vi "ui--test plot updates.vi"() -> ()   [LabVIEW 2021]
doc: "test the output of the theme on a graph and chart\n\n<b>Code Developed By:</b>\nTechnology Service Corporation\nwww.tsc.com/atcs\n\nDeveloper:\nDaniel Coons"
uses:
  <vilib>/numeric/Random Number (Range) DBL.vi
panel:
  out "Waveform Graph 2":dbl[][](graph)=[[0.13306085440791815, 0.0879688901503013, 0.036775389853692886, 0.6532669979114305, 0.08472829522034431, 0.9983087206518939, 0.7170974439775832, 0.09862926455924459, 0.9104404133169357, 0.0033720393869565157, 0.3438860221523703, 0.09569147282292523, 0.05190666424335655, 0.24694252161785646, 0.5168863730093075, 0.26831134492038067, 0.8230969685646516, 0.9814472257906978, 0.2272061024550942, 0.8098917477502172, 0.887589550084189, 0.6100626174511069, 0.96603126360236, 0.9151131295841366, 0.7482899830981327, 0.2780702935515085, 0.4086091237019789, 0.5812795207762955, 0.7774140578159758, 0.7741649634708238, 0.6857088358139753, 0.8553493754163002, 0.827686972367776, 0.2529298655163781, 0.4874874814367782, 0.5367329241411547, 0.41191999774024723, 0.9360704793200025, 0.8481368597935868, 0.5851233104174891, 0.7460626166357829, 0.7675282163169203, 0.5941383079043361, 0.6084437811903307, 0.9137270207566848, 0.14164206553644543, 0.944367703009636, 0.9882229095650765, 0.12807404389957888, 0.10166795257813277, 0.32112247869774735, 0.5621551625675485, 0.7091308394444604, 0.6473377689678865, 0.007821979537185886, 0.8113619812952195, 0.8073576350852725, 0.08930872921975874, 0.14986848733562108, 0.011921153237574034, 0.570553517421061, 0.377967728590463, 0.04482355518779935, 0.3186424001717114, 0.21330456282949317, 0.0454940725453894, 0.5821532512218817, 0.15991602882719103, 0.5719089521252518, 0.7776511172742474, 0.4787019383389124, 0.09976918045663452, 0.18257053533382273, 0.5464087033728721, 0.7482146674486345, 0.7493376528505136, 0.8963704778416384, 0.7063016502139434, 0.15944801725401514, 0.847500088853314, 0.17171175112658021, 0.14952470286069142, 0.15221036496154827, 0.10203582642171849, 0.6420353678306143, 0.4906006710065236, 0.2651490386034048, 0.06996255442612176, 0.4658855102620627, 0.5430459637216143, 0.744480966535523, 0.027436968629737102, 0.2562650988536652, 0.25014985041664684, 0.1804990531180204, 0.6957082808752657, 0.41848772122628874, 0.24793827529423518, 0.8451613763305086, 0.27204098993248893], [2.250567331065164, 2.155222595371875, 2.2912157636499053, 2.635194602081454, 2.0113751602913768, 2.7614535130644526, 2.192032474109693, 2.5440494750975704, 2.648149659054945, 2.4445680167950696, 2.216467853336293, 2.873700551200666, 2.082048417331531, 2.2564812644354224, 2.8276488760055103, 2.9029889347562903, 2.8000502636985525, 2.91643317675736, 2.9143263543098397, 2.018791563346438, 2.6447330992967113, 2.6591634333013783, 2.4422995021207727, 2.0507560523333925, 2.173974032844874, 2.0288400085476557, 2.736724222763875, 2.1594821423701753, 2.0884083642674853, 2.8437861581589017, 2.594905434692701, 2.9347939796818974, 2.797010298982248, 2.838478616946964, 2.0922518479967467, 2.6792853998702864, 2.5806796594219388, 2.5448755148190525, 2.3108227152712626, 2.4064380465081867, 2.881604687835967, 2.714153992346757, 2.7246345204675757, 2.4243597077332093, 2.835019087795636, 2.270228963400438, 2.5960929706836136, 2.6103082395488344, 2.246713305265933, 2.8016727933932177, 2.6836522256158846, 2.7676715761544943, 2.5088609150855046, 2.833814463085586, 2.037261950133102, 2.172913750388174, 2.6799708264242232, 2.7261659186713683, 2.7907715793753978, 2.270056703628074, 2.1145965797927166, 2.4016299344465812, 2.7153923091565155, 2.697971848331286, 2.1528446488866724, 2.084300506148895, 2.568400382123264, 2.9386149520700435, 2.1939145151262327, 2.943952377395883, 2.983422001711612, 2.437248724982225, 2.2088362783546343, 2.1457960347587344, 2.3722161277240112, 2.1723367223237133, 2.8712174085129925, 2.739840050537141, 2.1095238091832718, 2.8280621934872836, 2.994603810175076, 2.386886255698057, 2.9271371527505994, 2.020264802139174, 2.824470421902975, 2.13359228919213, 2.1597821381491773, 2.073776108944073, 2.22807338326564, 2.295848234568496, 2.2125822279768297, 2.695113663298697, 2.4618785516657646, 2.8260983836407716, 2.999201599112868, 2.8214814991913215, 2.419470908839876, 2.1521324775244146, 2.5721122929183666, 2.4514486019752018], [4.089061512326259, 4.647856745968412, 4.309407547794906, 4.560693965671817, 4.4312086267049935, 4.129245276854574, 4.0757929241775415, 4.609463902047546, 4.502170994575387, 4.873909478527954, 4.760370156932646, 4.04233179736546, 4.874324516259313, 4.298017859856133, 4.068046001412084, 4.739173641547795, 4.284737302487426, 4.008952794485126, 4.641819408684622, 4.798248059761852, 4.149623437648065, 4.55672454485615, 4.56122580169094, 4.091490230887189, 4.077975061044493, 4.752659198648686, 4.799909138524143, 4.007389112041125, 4.2607762424738365, 4.279512172714826, 4.431972417905556, 4.878454377380534, 4.206713125609022, 4.637365361432308, 4.7047035025037705, 4.445231353000265, 4.704813450576933, 4.68521120644791, 4.442092844866053, 4.141600078389089, 4.812990680788384, 4.530186859717628, 4.873307498467851, 4.878607714170448, 4.951439301914075, 4.287098614064677, 4.838307311467582, 4.754170250768442, 4.449630032859311, 4.427099315748594, 4.076858732914548, 4.5718517548709485, 4.820897116374338, 4.879501968144262, 4.096092007895505, 4.041306843528772, 4.828094156934113, 4.176532319160941, 4.355362756318517, 4.441429396646901, 4.978668176640304, 4.9833447914350035, 4.3664971395174055, 4.071166896356559, 4.937511757198768, 4.398521861278258, 4.363808490445537, 4.785504674454747, 4.202764875341174, 4.981895837134688, 4.564630482035177, 4.276113035945995, 4.592349279866313, 4.682836487325543, 4.4558409807445365, 4.157384709487678, 4.20593029948618, 4.678119867553962, 4.1005872997291135, 4.304906070497591, 4.160271840614688, 4.771275600453864, 4.846711403673545, 4.138674134279798, 4.775371171961872, 4.879827795522486, 4.46007662301777, 4.640085026025885, 4.692818233795106, 4.395254663053901, 4.0980676384603925, 4.660850995865211, 4.452635887216484, 4.146158353201239, 4.267302674967995, 4.36473064625353, 4.3939083058149, 4.240157204969512, 4.596736952450634, 4.3411290072014], [6.1350875737406705, 6.96390067748218, 6.296236534628202, 6.946318472784656, 6.943523884534723, 6.601285544937482, 6.873947587362833, 6.528168307104193, 6.2961921064669, 6.861032486602556, 6.807955384667905, 6.369341342223043, 6.8841669660414215, 6.457986003420221, 6.536993573697588, 6.226397028311644, 6.327944868701882, 6.583830979917187, 6.72295978337592, 6.518452734937067, 6.740960853531897, 6.237374648453478, 6.617995862253228, 6.959059327132556, 6.901659569927906, 6.980165277216955, 6.442029859519084, 6.618892236380024, 6.341076389768428, 6.486218024773717, 6.464373016931484, 6.79768621642226, 6.055827337472323, 6.668725224163492, 6.7599022048828905, 6.8361721482919515, 6.684921763655367, 6.092174934680624, 6.7671358035982045, 6.9861945722142895, 6.591252815685937, 6.05585383312341, 6.082373125493186, 6.376006437005647, 6.355758045934598, 6.389601506203173, 6.283552922181501, 6.299316751875152, 6.835130218092927, 6.710718281915929, 6.037532908874011, 6.120929381167479, 6.413251213480501, 6.876384155380969, 6.105135416990386, 6.361041627707308, 6.357576844723975, 6.4336242145227125, 6.67345081874056, 6.6236173179103295, 6.8805446728121105, 6.792790969573675, 6.096223330073096, 6.738982847223758, 6.754747110412485, 6.631242162144325, 6.696642255298795, 6.294476186559473, 6.274772493976961, 6.060436227809027, 6.122913049357602, 6.928403020909258, 6.648728225352519, 6.591089386786886, 6.732138174573499, 6.119587443147832, 6.300918299911057, 6.079794517108559, 6.778719366048897, 6.284692268755336, 6.004228810299407, 6.373199053484472, 6.222884782956066, 6.793173335340841, 6.1943750574246605, 6.793253335116867, 6.373811128014411, 6.058171148894061, 6.787745439297842, 6.816404253677163, 6.281272313817218, 6.385062702145819, 6.691809486812462, 6.247887741952185, 6.167846639456895, 6.003268291582449, 6.458997749826933, 6.675921521983426, 6.135774370297438, 6.573545193322419]] caption="Waveform Graph"
  out "Digital Waveform Graph":digitaldata(graph)
  out "XY Graph":cluster{i32[], dbl[]}[](graph)
  out "Waveform Chart 2":T1(graph)={"number: 0 to 1"=0.21847806490734922, "number: 0 to 1"=2.7228787825534773, "number: 0 to 1"=4.940418092061217, "number: 0 to 1"=6.187035254507957} caption="Waveform Chart"
  out "Waveform Graph":dbl[][](graph)=[[0.13306085440791815, 0.0879688901503013, 0.036775389853692886, 0.6532669979114305, 0.08472829522034431, 0.9983087206518939, 0.7170974439775832, 0.09862926455924459, 0.9104404133169357, 0.0033720393869565157, 0.3438860221523703, 0.09569147282292523, 0.05190666424335655, 0.24694252161785646, 0.5168863730093075, 0.26831134492038067, 0.8230969685646516, 0.9814472257906978, 0.2272061024550942, 0.8098917477502172, 0.887589550084189, 0.6100626174511069, 0.96603126360236, 0.9151131295841366, 0.7482899830981327, 0.2780702935515085, 0.4086091237019789, 0.5812795207762955, 0.7774140578159758, 0.7741649634708238, 0.6857088358139753, 0.8553493754163002, 0.827686972367776, 0.2529298655163781, 0.4874874814367782, 0.5367329241411547, 0.41191999774024723, 0.9360704793200025, 0.8481368597935868, 0.5851233104174891, 0.7460626166357829, 0.7675282163169203, 0.5941383079043361, 0.6084437811903307, 0.9137270207566848, 0.14164206553644543, 0.944367703009636, 0.9882229095650765, 0.12807404389957888, 0.10166795257813277, 0.32112247869774735, 0.5621551625675485, 0.7091308394444604, 0.6473377689678865, 0.007821979537185886, 0.8113619812952195, 0.8073576350852725, 0.08930872921975874, 0.14986848733562108, 0.011921153237574034, 0.570553517421061, 0.377967728590463, 0.04482355518779935, 0.3186424001717114, 0.21330456282949317, 0.0454940725453894, 0.5821532512218817, 0.15991602882719103, 0.5719089521252518, 0.7776511172742474, 0.4787019383389124, 0.09976918045663452, 0.18257053533382273, 0.5464087033728721, 0.7482146674486345, 0.7493376528505136, 0.8963704778416384, 0.7063016502139434, 0.15944801725401514, 0.847500088853314, 0.17171175112658021, 0.14952470286069142, 0.15221036496154827, 0.10203582642171849, 0.6420353678306143, 0.4906006710065236, 0.2651490386034048, 0.06996255442612176, 0.4658855102620627, 0.5430459637216143, 0.744480966535523, 0.027436968629737102, 0.2562650988536652, 0.25014985041664684, 0.1804990531180204, 0.6957082808752657, 0.41848772122628874, 0.24793827529423518, 0.8451613763305086, 0.27204098993248893], [2.250567331065164, 2.155222595371875, 2.2912157636499053, 2.635194602081454, 2.0113751602913768, 2.7614535130644526, 2.192032474109693, 2.5440494750975704, 2.648149659054945, 2.4445680167950696, 2.216467853336293, 2.873700551200666, 2.082048417331531, 2.2564812644354224, 2.8276488760055103, 2.9029889347562903, 2.8000502636985525, 2.91643317675736, 2.9143263543098397, 2.018791563346438, 2.6447330992967113, 2.6591634333013783, 2.4422995021207727, 2.0507560523333925, 2.173974032844874, 2.0288400085476557, 2.736724222763875, 2.1594821423701753, 2.0884083642674853, 2.8437861581589017, 2.594905434692701, 2.9347939796818974, 2.797010298982248, 2.838478616946964, 2.0922518479967467, 2.6792853998702864, 2.5806796594219388, 2.5448755148190525, 2.3108227152712626, 2.4064380465081867, 2.881604687835967, 2.714153992346757, 2.7246345204675757, 2.4243597077332093, 2.835019087795636, 2.270228963400438, 2.5960929706836136, 2.6103082395488344, 2.246713305265933, 2.8016727933932177, 2.6836522256158846, 2.7676715761544943, 2.5088609150855046, 2.833814463085586, 2.037261950133102, 2.172913750388174, 2.6799708264242232, 2.7261659186713683, 2.7907715793753978, 2.270056703628074, 2.1145965797927166, 2.4016299344465812, 2.7153923091565155, 2.697971848331286, 2.1528446488866724, 2.084300506148895, 2.568400382123264, 2.9386149520700435, 2.1939145151262327, 2.943952377395883, 2.983422001711612, 2.437248724982225, 2.2088362783546343, 2.1457960347587344, 2.3722161277240112, 2.1723367223237133, 2.8712174085129925, 2.739840050537141, 2.1095238091832718, 2.8280621934872836, 2.994603810175076, 2.386886255698057, 2.9271371527505994, 2.020264802139174, 2.824470421902975, 2.13359228919213, 2.1597821381491773, 2.073776108944073, 2.22807338326564, 2.295848234568496, 2.2125822279768297, 2.695113663298697, 2.4618785516657646, 2.8260983836407716, 2.999201599112868, 2.8214814991913215, 2.419470908839876, 2.1521324775244146, 2.5721122929183666, 2.4514486019752018], [4.089061512326259, 4.647856745968412, 4.309407547794906, 4.560693965671817, 4.4312086267049935, 4.129245276854574, 4.0757929241775415, 4.609463902047546, 4.502170994575387, 4.873909478527954, 4.760370156932646, 4.04233179736546, 4.874324516259313, 4.298017859856133, 4.068046001412084, 4.739173641547795, 4.284737302487426, 4.008952794485126, 4.641819408684622, 4.798248059761852, 4.149623437648065, 4.55672454485615, 4.56122580169094, 4.091490230887189, 4.077975061044493, 4.752659198648686, 4.799909138524143, 4.007389112041125, 4.2607762424738365, 4.279512172714826, 4.431972417905556, 4.878454377380534, 4.206713125609022, 4.637365361432308, 4.7047035025037705, 4.445231353000265, 4.704813450576933, 4.68521120644791, 4.442092844866053, 4.141600078389089, 4.812990680788384, 4.530186859717628, 4.873307498467851, 4.878607714170448, 4.951439301914075, 4.287098614064677, 4.838307311467582, 4.754170250768442, 4.449630032859311, 4.427099315748594, 4.076858732914548, 4.5718517548709485, 4.820897116374338, 4.879501968144262, 4.096092007895505, 4.041306843528772, 4.828094156934113, 4.176532319160941, 4.355362756318517, 4.441429396646901, 4.978668176640304, 4.9833447914350035, 4.3664971395174055, 4.071166896356559, 4.937511757198768, 4.398521861278258, 4.363808490445537, 4.785504674454747, 4.202764875341174, 4.981895837134688, 4.564630482035177, 4.276113035945995, 4.592349279866313, 4.682836487325543, 4.4558409807445365, 4.157384709487678, 4.20593029948618, 4.678119867553962, 4.1005872997291135, 4.304906070497591, 4.160271840614688, 4.771275600453864, 4.846711403673545, 4.138674134279798, 4.775371171961872, 4.879827795522486, 4.46007662301777, 4.640085026025885, 4.692818233795106, 4.395254663053901, 4.0980676384603925, 4.660850995865211, 4.452635887216484, 4.146158353201239, 4.267302674967995, 4.36473064625353, 4.3939083058149, 4.240157204969512, 4.596736952450634, 4.3411290072014], [6.1350875737406705, 6.96390067748218, 6.296236534628202, 6.946318472784656, 6.943523884534723, 6.601285544937482, 6.873947587362833, 6.528168307104193, 6.2961921064669, 6.861032486602556, 6.807955384667905, 6.369341342223043, 6.8841669660414215, 6.457986003420221, 6.536993573697588, 6.226397028311644, 6.327944868701882, 6.583830979917187, 6.72295978337592, 6.518452734937067, 6.740960853531897, 6.237374648453478, 6.617995862253228, 6.959059327132556, 6.901659569927906, 6.980165277216955, 6.442029859519084, 6.618892236380024, 6.341076389768428, 6.486218024773717, 6.464373016931484, 6.79768621642226, 6.055827337472323, 6.668725224163492, 6.7599022048828905, 6.8361721482919515, 6.684921763655367, 6.092174934680624, 6.7671358035982045, 6.9861945722142895, 6.591252815685937, 6.05585383312341, 6.082373125493186, 6.376006437005647, 6.355758045934598, 6.389601506203173, 6.283552922181501, 6.299316751875152, 6.835130218092927, 6.710718281915929, 6.037532908874011, 6.120929381167479, 6.413251213480501, 6.876384155380969, 6.105135416990386, 6.361041627707308, 6.357576844723975, 6.4336242145227125, 6.67345081874056, 6.6236173179103295, 6.8805446728121105, 6.792790969573675, 6.096223330073096, 6.738982847223758, 6.754747110412485, 6.631242162144325, 6.696642255298795, 6.294476186559473, 6.274772493976961, 6.060436227809027, 6.122913049357602, 6.928403020909258, 6.648728225352519, 6.591089386786886, 6.732138174573499, 6.119587443147832, 6.300918299911057, 6.079794517108559, 6.778719366048897, 6.284692268755336, 6.004228810299407, 6.373199053484472, 6.222884782956066, 6.793173335340841, 6.1943750574246605, 6.793253335116867, 6.373811128014411, 6.058171148894061, 6.787745439297842, 6.816404253677163, 6.281272313817218, 6.385062702145819, 6.691809486812462, 6.247887741952185, 6.167846639456895, 6.003268291582449, 6.458997749826933, 6.675921521983426, 6.135774370297438, 6.573545193322419]]
  out "Waveform Chart":T1(graph)={"number: 0 to 1"=0.21847806490734922, "number: 0 to 1"=2.7228787825534773, "number: 0 to 1"=4.940418092061217, "number: 0 to 1"=6.187035254507957}
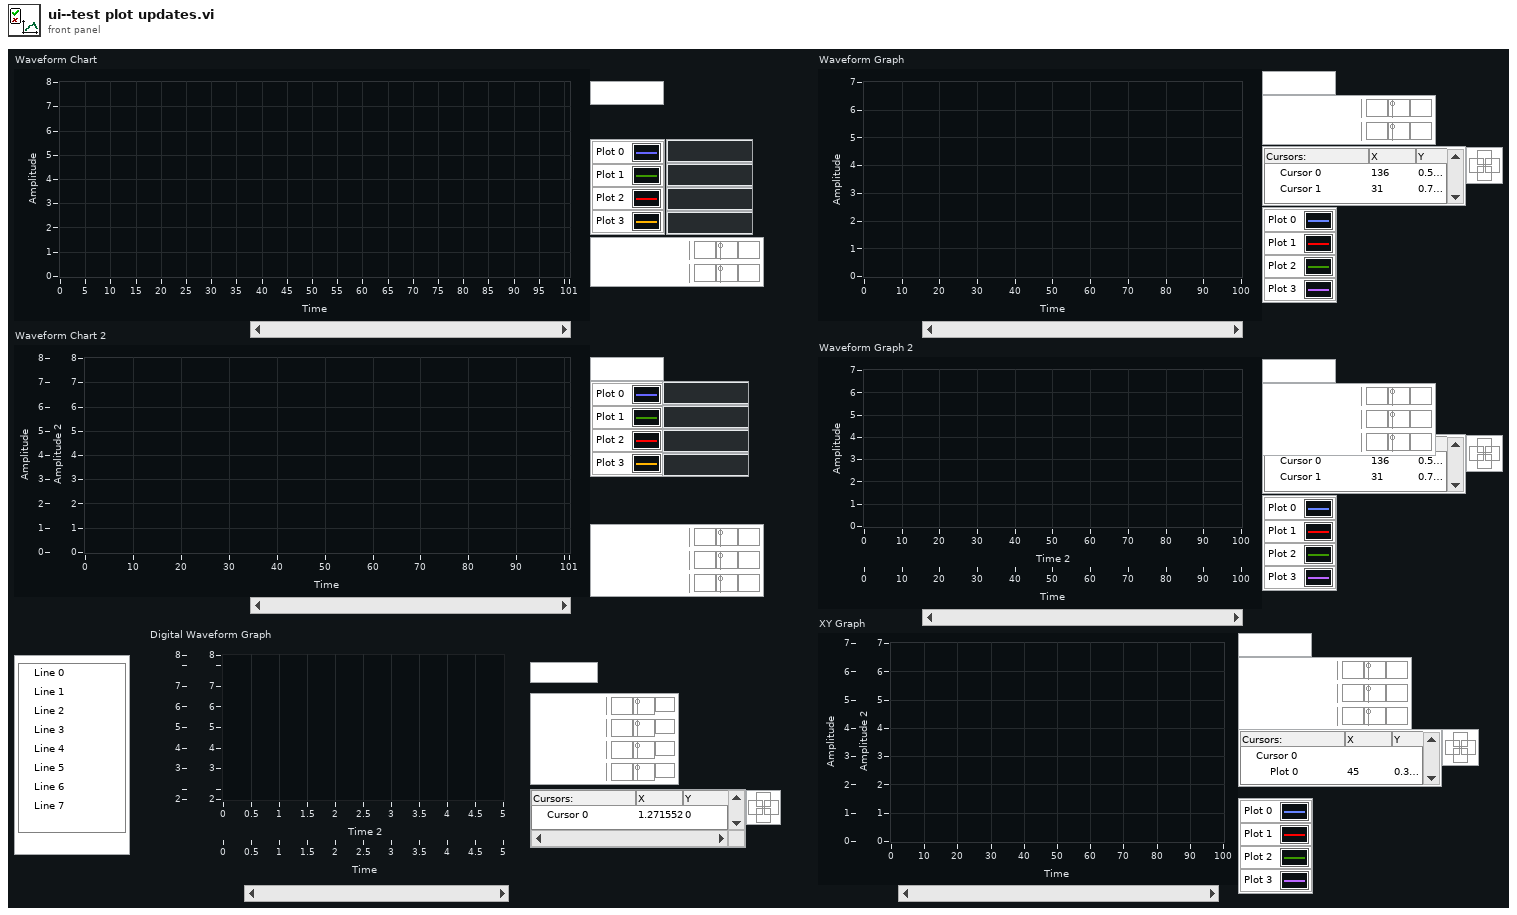
[diagram p1: front panel]
types:
  T1 = cluster{"number: 0 to 1":dbl, "number: 0 to 1":dbl, "number: 0 to 1":dbl, "number: 0 to 1":dbl}
  T2 = cluster{"number: 0 to 1":dbl, "number: 0 to 1":dbl, "number: 0 to 1":dbl, "number: 0 to 1":dbl}[]
  T3 = cluster{"number: 0 to 1":dbl, "number":dbl, "number":dbl, "number":dbl}
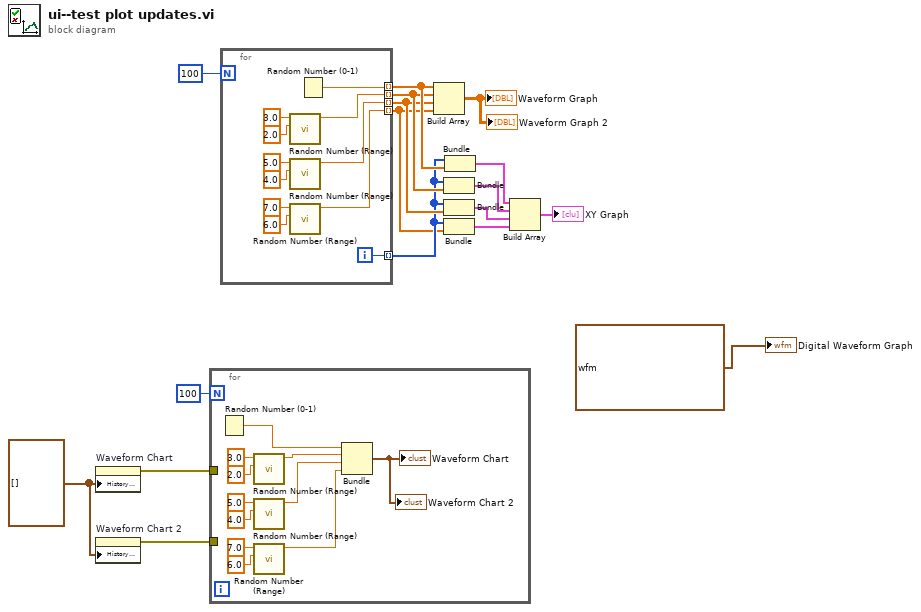
[diagram p0: block diagram]
diagram:
  w2 = T2 [] ("History Data")
  n1 = property on="Waveform Chart" class="WFChart (strict)"("History Data"=w2) -> (error out=w15:errorcluster)  [unwired: 2 in, 1 out]
  n2 = property on="Waveform Chart 2" class="WFChart (strict)"("History Data"=w2) -> (error out=w1:errorcluster)  [unwired: 2 in, 1 out]
  n3 = for {
    N: 100 -> [_]
    tunnel: w15 -> [_]
    tunnel: w1 -> [_]
    n4 = Random Number (0-1)() -> (number: 0 to 1=w28:dbl)
    n5 = call-poly <vilib>:"Random Number (Range).vi"("lower bound (0)"=2.0, "upper bound (100)"=3.0) -> ("number"=w25:dbl)  [unwired: 9 in]
    n6 = call-poly <vilib>:"Random Number (Range).vi"("lower bound (0)"=4.0, "upper bound (100)"=5.0) -> ("number"=w19:dbl)  [unwired: 9 in]
    n7 = call-poly <vilib>:"Random Number (Range).vi"("lower bound (0)"=6.0, "upper bound (100)"=7.0) -> ("number"=w20:dbl)  [unwired: 9 in]
    n8 = Bundle("number: 0 to 1"=w28, "number"=w25, "number"=w19, "number"=w20) -> (→"Waveform Chart" →"Waveform Chart 2":T3)  [unwired: 1 in]
  }
  n9 = for {
    N: 100 -> [_]
    tunnel: [w39] -> w14 mode=indexing
    tunnel: [w32] -> w10 mode=indexing
    tunnel: [w31] -> w9 mode=indexing
    tunnel: [w30] -> w6 mode=indexing
    tunnel: [w29] -> w7 mode=indexing
    i -> [w29]
    n10 = call-poly <vilib>:"Random Number (Range).vi"("lower bound (0)"=2.0, "upper bound (100)"=3.0) -> ("number"=w32:dbl)  [unwired: 9 in]
    n11 = call-poly <vilib>:"Random Number (Range).vi"("lower bound (0)"=4.0, "upper bound (100)"=5.0) -> ("number"=w31:dbl)  [unwired: 9 in]
    n12 = call-poly <vilib>:"Random Number (Range).vi"("lower bound (0)"=6.0, "upper bound (100)"=7.0) -> ("number"=w30:dbl)  [unwired: 9 in]
    n13 = Random Number (0-1)() -> (number: 0 to 1=w39:dbl)
  }
  n14 = Build Array(w14, w10, w9, w6) -> (→"Waveform Graph" →"Waveform Graph 2":dbl[][])
  n15 = Bundle(w7, w10) -> (w11:cluster{i32[], dbl[]})  [unwired: 1 in]
  n16 = Bundle(w7, w9) -> (w8:cluster{i32[], dbl[]})  [unwired: 1 in]
  n17 = Bundle(w7, w6) -> (w5:cluster{i32[], dbl[]})  [unwired: 1 in]
  n18 = Bundle(w7, w14) -> (w13:cluster{i32[], dbl[]})  [unwired: 1 in]
  n19 = Build Array(w13, w11, w8, w5) -> (→"XY Graph":cluster{i32[], dbl[]}[])
  "Digital Waveform Graph" <- digitaldata {"transitions"=[], "data"=[[0, 0, 0, 0, 0, 0, 1, 0], [0, 0, 0, 0, 0, 1, 1, 1], [0, 0, 0, 0, 0, 1, 0, 0], [0, 0, 1, 0, 1, 1, 0, 1], [1, 1, 1, 1, 1, 1, 1, 1]]} ("Digital Data")
